vi "Datum-Uhrzeit-Cluster nach Zeitstempel.vi"(1 "Datum/Zeit":T1) -> (0 "Zeitstempel":timestamp)   [LabVIEW 2020, in "FT-IR.lvlib" / "TOOLweb Interface.lvlib" / "TOOLweb Interface Hilfs-VIs.lvlib"]
doc: "Formt den Datum/Zeit-Cluster in einen korrekten Zeitstempel um."
uses:
  TOOLweb Interface Hilfs-VIs.lvlib
  <vilib>/Utility/miscctls.llb/LVDateTimeRec.ctl
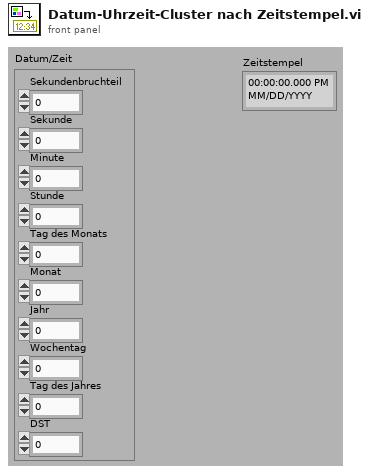
[diagram p1: front panel]
types:
  T1 = typedef "LVDateTimeRec.ctl" = cluster{"fractional second":dbl, "second":i32, "minute":i32, "hour":i32, "day of month":i32, "month":i32, "year":i32, "day of week":i32, "day of year":i32, "DST":i32}
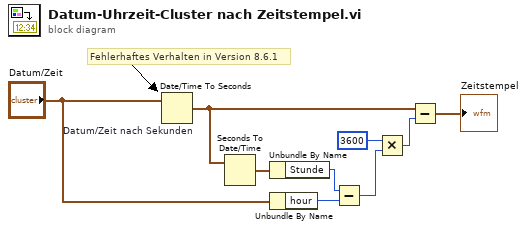
[diagram p0: block diagram]
diagram:
  # "Fehlerhaftes Verhalten in Version 8.6.1"
  n1 = Date/Time To Seconds "Datum/Zeit nach Sekunden"(2:"Datum/Zeit") -> (0:w6:timestamp)  [unwired: 1 out]
  n2 = Seconds To Date/Time(time stamp (now)=w6) -> (date time rec=w9:T1)  [unwired: 1 out]
  n3 = Unbundle By Name(w9) -> ("Stunde"=w8:i32)
  n4 = Unbundle By Name("Datum/Zeit") -> ("hour"=w7:i32)
  n5 = Subtract(x=w8, y=w7) -> (x-y=w3:i32)
  n6 = Multiply(x=3600 ("y"), y=w3) -> (x*y=w2:i32)
  n7 = Subtract(x=w6, y=w2) -> (x-y=→"Zeitstempel":timestamp)
